vi "Number of Frequency Components.vi"(0 "MRN in":refnum<class "Moving Ripple Noise.lvclass">, 11 "error in (no error)":errorcluster) -> (4 "MRN out":refnum<class "Moving Ripple Noise.lvclass">, 8 "Nfreq":i32, 15 "error out":errorcluster)   [LabVIEW 2015, in "Moving Ripple Noise.lvclass"]
uses:
  Moving Ripple Noise.lvclass
  Moving Ripple Noise.lvclass/Moving Ripple Noise.ctl
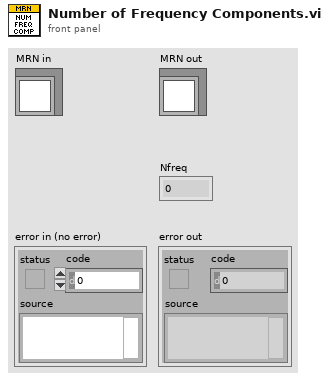
[diagram p1: front panel]
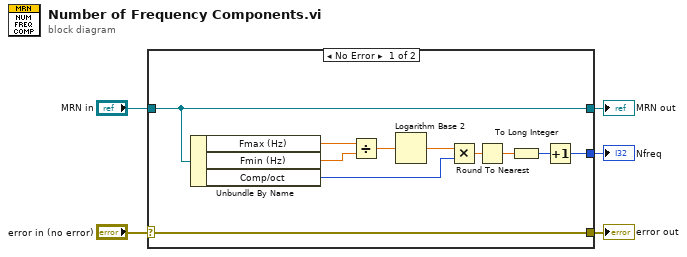
[diagram p0: block diagram]
diagram:
  n1 = case shown="No Error" "error in (no error)" {
    selector: "error in (no error)" -> [w16 w18]
    tunnel: [w16 w18] -> w4
    tunnel: [w7 w17] -> w2
    tunnel: "MRN in" -> [w7 w17]
    tunnel: [w6 _] -> w1
    frame No Error {
      n2 = Unbundle By Name(w7) -> ("Fmax (Hz)"=w15:dbl, "Fmin (Hz)"=w8:dbl, "Comp/oct"=w9:i32)
      n3 = Divide(x=w15, y=w8) -> (x/y=w14:dbl)
      n4 = Logarithm Base 2(1:w14) -> (0:w13:dbl)
      n5 = Multiply(x=w13, y=w9) -> (x*y=w12:dbl)
      n6 = Round To Nearest(number=w12) -> (nearest integer value=w10:dbl)
      n7 = To Long Integer(number=w10) -> (32bit integer=w11:i32)
      n8 = Increment(x=w11) -> (x+1=w6:i32)
    }
    frame Error {
    }
  }
  "error out" <- w4
  "MRN out" <- w2
  "Nfreq" <- w1
